vi "Read Edit Time Configuration.vi"(8 "error in (no error)":errorcluster, 11 "Session in":refnum<class "Plugin Session.lvclass">) -> (0 "error out":errorcluster, 2 "Edit Time Configuration":string, 3 "Session out":refnum<class "Plugin Session.lvclass">)   [LabVIEW 2021, in "InstrumentStudio Plugin SDK.lvlib" / "Plugin Session.lvclass"]
doc: "Call this VI to read the edit-time configuration string for your plugin panel."
uses:
  Plugin Session.lvclass
  Plugin Session.lvclass/Plugin Session.ctl
  Read Session Id.vi
  NationalInstruments.VIHost.Interop.dll
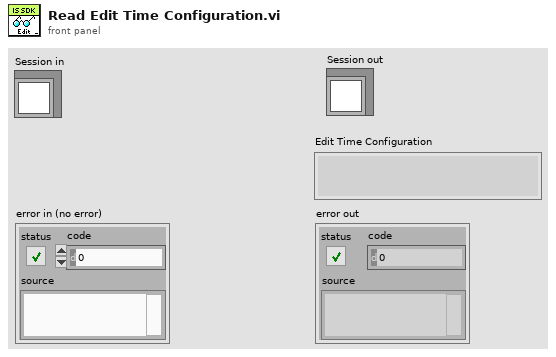
[diagram p1: front panel]
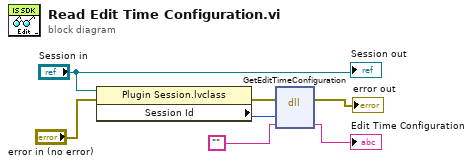
[diagram p0: block diagram]
diagram:
  n1 = property class="Plugin Session.lvclass"(reference="Session in", error in="error in (no error)") -> (error out=w2:errorcluster, "Session Id"=w6:u64)  [unwired: 1 out]
  n2 = dll-call lib="C:/git/srd-adg-rf/dst/dstd/DSTInstStudio/source/utilities/PluginSDK/NationalInstruments.VIHost.Interop.dll" fn="GetEditTimeConfiguration"(error in=w2, "hostId"=w6, "configuration"="") -> (error out=→"error out":errorcluster, "configuration"=→"Edit Time Configuration":string)  [unwired: 4 in, 1 out]
  "Session out" <- "Session in"
